vi "getContext.vi"(11 "Controller in":refnum<class "Controller.lvclass">) -> (2 "Context":refnum<class "Context.lvclass">, 3 "Controller out":refnum<class "Controller.lvclass">)   [LabVIEW 2016, in "Controller.lvclass"]
uses:
  Controller.lvclass
  Context/Context/Context.lvclass
  Controller.lvclass/Controller.ctl
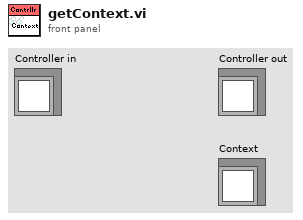
[diagram p1: front panel]
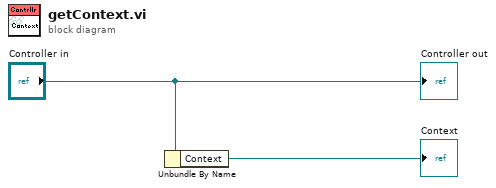
[diagram p0: block diagram]
diagram:
  n1 = Unbundle By Name("Controller in") -> ("Context"=→"Context":refnum<class "Context.lvclass">)
  "Controller out" <- "Controller in"
